vi "Setup.vi"(8 "error in (no error)":errorcluster, 9 "Str Refnum":refnum<vi>, 10 "VI Reference":refnum<vi>, 11 "Dialog in":refnum<class "Dialog.lvclass">) -> (0 "error out":errorcluster, 2 "VI reference (dup)":refnum<vi>, 3 "Dialog out":refnum<class "Dialog.lvclass">)   [LabVIEW 2012, in "Dialog.lvlib" / "Dialog.lvclass"]
uses:
  Dialog.lvclass
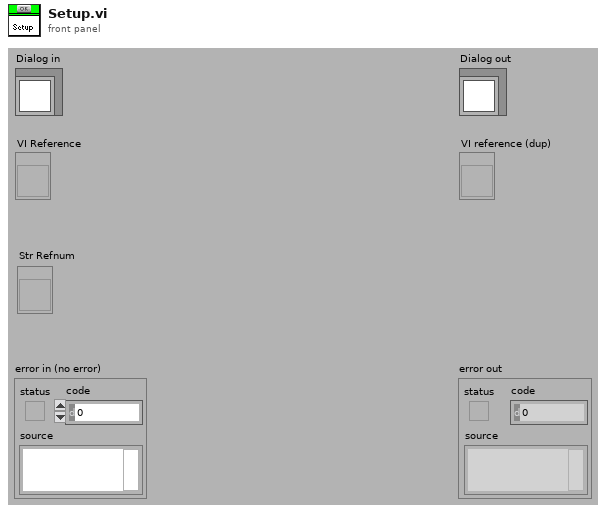
[diagram p1: front panel]
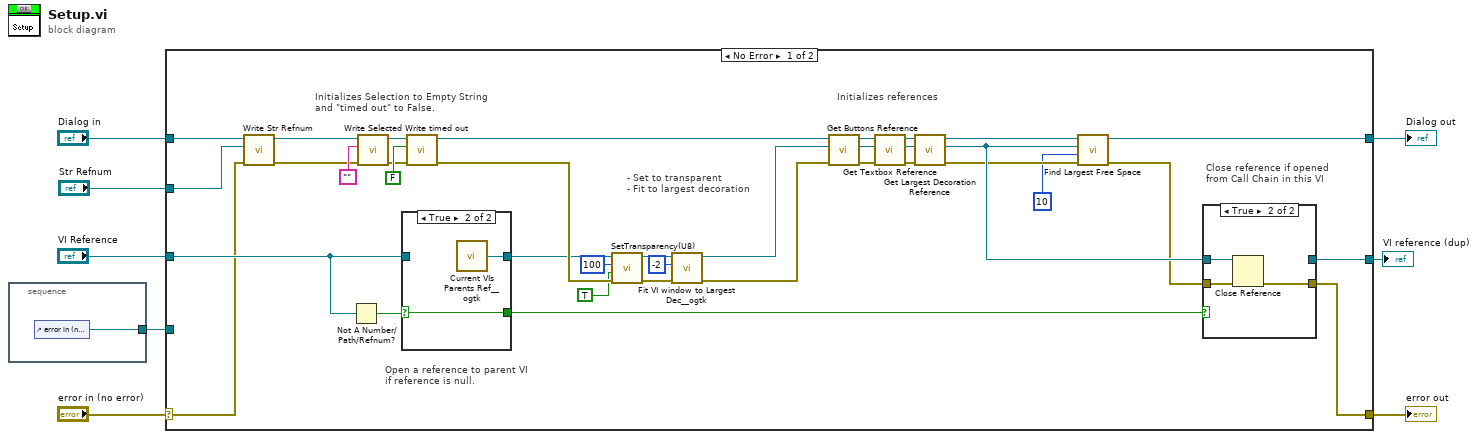
[diagram p0: block diagram]
diagram:
  n1 = stacked-sequence {
    tunnel: [w9] -> w1
    frame #0 {
      n2 = control-ref of="error in (no error)"() -> (w9:refnum<vi>)
    }
  }
  n3 = case shown="No Error" "error in (no error)" {
    selector: "error in (no error)" -> [w17 w57]
    tunnel: [w24 w57] -> w7
    tunnel: [w13 w56] -> w5
    tunnel: "Dialog in" -> [w19 w56]
    tunnel: "VI Reference" -> [w28 w55]
    tunnel: [w25 w55] -> w3
    tunnel: "Str Refnum" -> [w20 _]
    tunnel: w1 -> [_ _]
    frame No Error {
      # "Open a reference to parent VI\nif reference is null."
      # "Close reference if opened\nfrom Call Chain in this VI"
      # "Initializes references"
      # "Initializes Selection to Empty String\nand \"timed out\" to False."
      # "- Set to transparent\n- Fit to largest decoration"
      n4 = call-dynamic "Write Str Refnum.vi"("error in (no error)"=w17, "Str Refnum"=w20, "Dialog.lvclass in"=w19) -> ("error out"=w16:errorcluster, "Dialog.lvclass out"=w18:refnum<class "Dialog.lvclass">)  [unwired: 7 out]
      n5 = Not A Number/Path/Refnum?(number/path/refnum=w28) -> (NaN/Path/Refnum?=w29:bool)
      n6 = call-dynamic "Write Selected.vi"("error in (no error)"=w16, "Selected"="", "Dialog.lvclass in"=w18) -> ("error out"=w38:errorcluster, "Dialog.lvclass out"=w40:refnum<class "Dialog.lvclass">)  [unwired: 7 out]
      n7 = case shown="True" w29 {
        selector: w29 -> [w51 w53]
        tunnel: w28 -> [w52 _]
        tunnel: [w52 w54] -> w27
        tunnel: [w51 w53] -> w26
        frame False {
        }
        frame True {
          n8 = call <userlib>:"Current VIs Parents Ref__ogtk.vi"() -> ("Calling VI's Reference"=w54:refnum<vi>)  [unwired: 2 out]
        }
      }
      n9 = call-dynamic "Write timed out.vi"("error in (no error)"=w38, "timed out?"=FALSE, "Dialog.lvclass in"=w40) -> ("error out"=w30:errorcluster, "Dialog.lvclass out"=w31:refnum<class "Dialog.lvclass">)  [unwired: 7 out]
      n10 = call "SetTransparency(U8).vi"("error in"=w30, "Run VI Transparently (T)"=TRUE, "Transparency (%)"=u8 100, "VI Reference (calling VI)"=w27) -> ("error out"=w43:errorcluster, "dup VI Reference"=w42:refnum<vi>)  [unwired: 6 out]
      n11 = call <userlib>:"Fit VI window to Largest Dec__ogtk.vi"("error in (no error)"=w43, "border spacing (2 px)"=-2, "VI Ref (calling VI)"=w42) -> ("error out"=w21:errorcluster, "dup VI Ref"=w22:refnum<vi>)  [unwired: 3 out]
      n12 = call "Get Buttons Reference.vi"("error in (no error)"=w21, "VI reference (calling)"=w22, "Dialog in"=w31) -> ("error out"=w34:errorcluster, "VI reference (dup)"=w33:refnum<vi>, "Dialog out"=w35:refnum<class "Dialog.lvclass">)  [unwired: 6 out]
      n13 = call "Get Textbox Reference.vi"("error in (no error)"=w34, "VI reference (calling)"=w33, "Dialog in"=w35) -> ("error out"=w36:errorcluster, "VI reference (dup)"=w32:refnum<vi>, "Dialog out"=w37:refnum<class "Dialog.lvclass">)  [unwired: 6 out]
      n14 = call "Get Largest Decoration Reference.vi"("error in (no error)"=w36, "VI reference (calling)"=w32, "Dialog in"=w37) -> ("error out"=w12:errorcluster, "VI reference (dup)"=w15:refnum<vi>, "Dialog out"=w14:refnum<class "Dialog.lvclass">)  [unwired: 6 out]
      n15 = call-dynamic "Find Largest Free Space.vi"("error in (no error)"=w12, "border (10)"=i16 10 ("border (5)"), "VI reference"=w15, "Dialog in"=w14) -> ("error out"=w11:errorcluster, "Dialog out"=w13:refnum<class "Dialog.lvclass">)  [unwired: 6 out]
      n16 = case shown="True" w26 {
        tunnel: w15 -> [w47 w50]
        tunnel: [w47 _] -> w25
        tunnel: w11 -> [w46 w49]
        tunnel: [w46 w48] -> w24
        frame False {
        }
        frame True {
          n17 = Close Reference(reference=w50, error in (no error)=w49) -> (error out=w48:errorcluster)
        }
      }
    }
    frame Error {
    }
  }
  "error out" <- w7
  "Dialog out" <- w5
  "VI reference (dup)" <- w3
